vi "Read Sync.vi"(8 "error in (no error)":errorcluster, 11 "DAQmx-Bus in":refnum<class "DAQmx-Bus.lvclass">) -> (0 "error out":errorcluster, 2 "Sync":refnum<notifier>, 3 "DAQmx-Bus out":refnum<class "DAQmx-Bus.lvclass">)   [LabVIEW 2021, in "DAQmx-Bus.lvclass"]
uses:
  DAQmx-Bus.lvclass
  DAQmx-Bus.lvclass/DAQmx-Bus.ctl
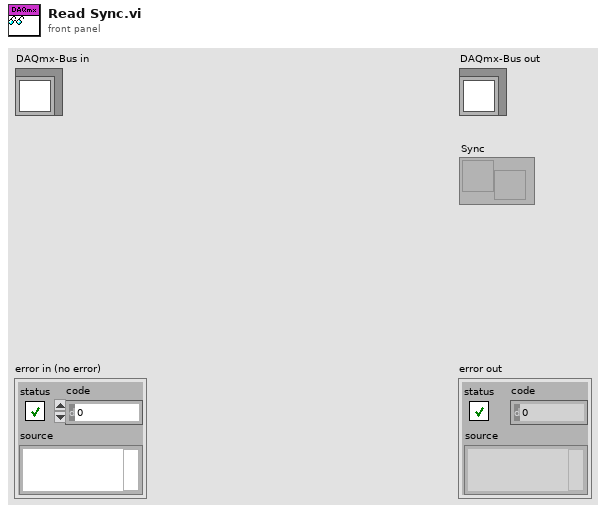
[diagram p1: front panel]
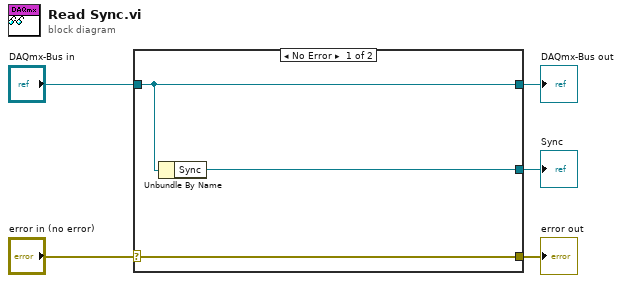
[diagram p0: block diagram]
diagram:
  n1 = case shown="No Error" "error in (no error)" {
    selector: "error in (no error)" -> [w8 w9]
    tunnel: [w8 w9] -> w4
    tunnel: [w7 w10] -> w2
    tunnel: "DAQmx-Bus in" -> [w7 w10]
    tunnel: [w6 _] -> w1
    frame No Error {
      n2 = Unbundle By Name(w7) -> ("Sync"=w6:refnum<notifier>)
    }
    frame Error {
    }
  }
  "error out" <- w4
  "DAQmx-Bus out" <- w2
  "Sync" <- w1
